vi "Vertical.vi"(0 "Instrument Handle In":i32, 1 "Coupling":i32(ring) items=["AC", "DC", "ACLFR"], 2 "Impedance":T1 items=["50 Ohm", "1M Ohm"], 5 "Channel":i32(ring) items=["Input Channel 1", "Input Channel 2", "Input Channel 3", "Input Channel 4"], 7 "Range":dbl, 9 "Offset":dbl, 11 "error in":errorcluster, 12 "Lowpass Filter":i32(ring) items=["Bypass", "Lowpass"], 13 "Attenuation":dbl) -> (4 "Instrument Handle Out":i32, 15 "error out":errorcluster)   [LabVIEW 8.6, in "ZTScopeM.lvlib"]
doc: "Configure the vertical settings for the selected channel"
uses:
  ZTScopeM.lvlib
  Impedance.ctl
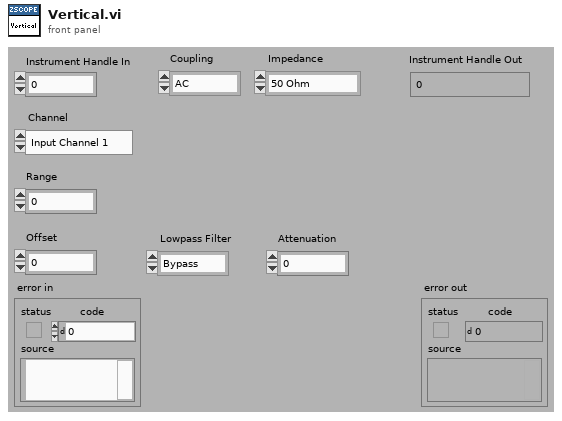
[diagram p1: front panel]
types:
  T1 = typedef "ZTScopeM.lvlib/Impedance.ctl" = dbl
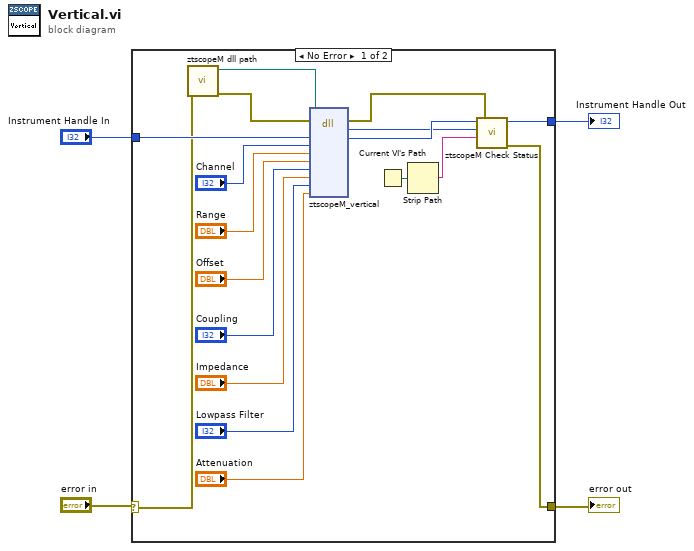
[diagram p0: block diagram]
diagram:
  n1 = case shown="No Error" "error in" {
    selector: "error in" -> [w8 w23]
    tunnel: [w10 w23] -> w2
    tunnel: "Instrument Handle In" -> [w22 w24]
    tunnel: [w9 w24] -> w3
    frame #0 {
      n2 = call "ztscopeM dll path.vi"("error in (no error)"=w8) -> ("error out"=w6:errorcluster, "<instrument>.dll path"=w7:path)  [unwired: 9 in]
      n3 = dll-call lib="C:/Program Files (x86)/National Instruments/LabVIEW 2013/instr.lib/ztscopem/ztscopeM.dll" fn="ztscopeM_vertical"(path in=w7, error in=w6, "instrumentHandle"=w22, "channel"="Channel", "range"="Range", "offset"="Offset", "coupling"="Coupling", "impedance"="Impedance", "lowpassFilter"="Lowpass Filter", "attenuation"="Attenuation") -> (error out=w5:errorcluster, w11:i32, "instrumentHandle"=w12:i32)  [unwired: 8 in, 1 out]
      n4 = Current VI's Path() -> (path=w14:path)
      n5 = Strip Path(path=w14) -> (name=w13:string)  [unwired: 1 out]
      n6 = call "ztscopeM Check Status.vi"("error in"=w5, "name of VI"=w13, "status (return code)"=w11, "instrument handle in"=w12) -> ("error out"=w10:errorcluster, "instrument handle out"=w9:i32)  [unwired: 2 in]
    }
    frame #1 {
    }
  }
  "Instrument Handle Out" <- w3
  "error out" <- w2
